vi "ListThisLevelDependencies.vi"(8 "error in (no error)":errorcluster, 11 "SMO in":refnum<class "SMO.lvclass">) -> (0 "error out":errorcluster, 2 "[My Dependencies]":refnum<class "SMO.lvclass">[](array[class]), 3 "SMO out":refnum<class "SMO.lvclass">)   [LabVIEW 2013, in "SMO.lvclass"]
uses:
  SMO.lvclass
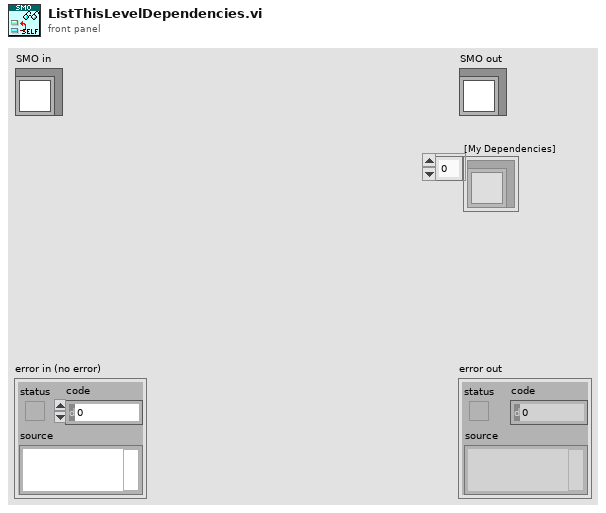
[diagram p1: front panel]
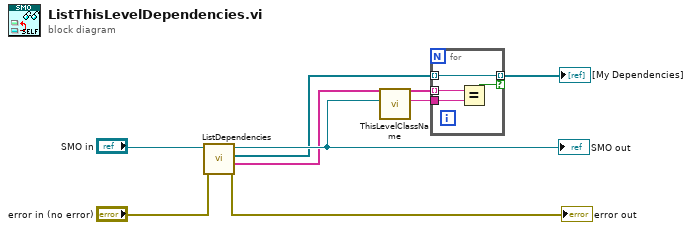
[diagram p0: block diagram]
diagram:
  n1 = call "ListDependencies.vi"("error in (no error)"="error in (no error)", "SMO in"="SMO in") -> ("error out"=→"error out":errorcluster, "Level"=w2:string[], "[Dependencies]"=w3:refnum<class "SMO.lvclass">[], "SMO out"=w5:refnum<class "SMO.lvclass">)  [unwired: 6 in]
  "SMO out" <- w5
  n2 = call "ThisLevelClassName.vi"("SMO"=w5) -> ("Level class name"=w1:string)  [unwired: 10 in]
  n3 = for {
    tunnel: [w12] -> w8 mode=indexing if=w11
    tunnel: w3 -> [w12] mode=indexing
    tunnel: w2 -> [w10] mode=indexing
    tunnel: w1 -> [w9]
    n4 = Equal?(x=w10, y=w9) -> (x = y?=w11:bool)
  }
  "[My Dependencies]" <- w8
